vi "input.vi"(8 "error in":errorcluster, 10 "input allocation":T1, 11 "BuckBoost runtime in":refnum<class "BuckBoost runtime.lvclass">) -> (0 "error out":errorcluster, 2 "input data":T1, 3 "BuckBoost runtime out":refnum<class "BuckBoost runtime.lvclass">)   [LabVIEW 2017, in "BuckBoost runtime.lvclass"]
doc: "Provides an interface for reading data from a module at runtime. While this interface performs no operations, a child should provide an override which may read from any open sessions, references, or interfaces."
uses:
  BuckBoost runtime.lvclass
  <vilib>/NI/Tag Bus/table/data table.ctl
  input user data.ctl
  BuckBoost runtime.lvclass/BuckBoost runtime.ctl
  <vilib>/NI/PowerElectronicsControl/Buck-Boost/RealTime/BuckBoostInterface.lvlib
  <vilib>/NI/Tag Bus/table/data table.lvlib
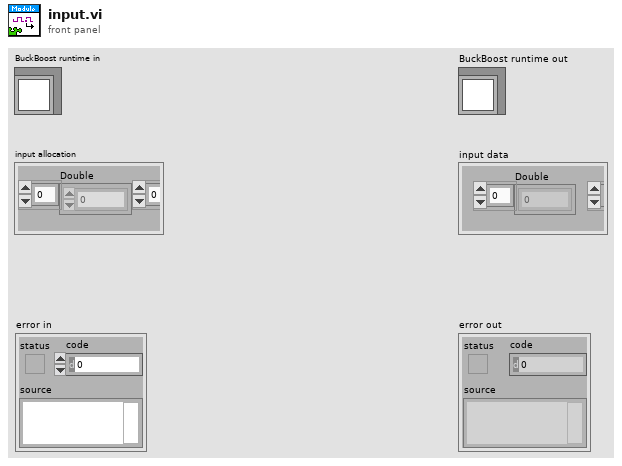
[diagram p1: front panel]
types:
  T1 = typedef "tag bus.lvlib/data table.lvlib/data table.ctl" = cluster{"Double":dbl[], "Single":sgl[], "I64":i64[], "I32":i32[], "I16":i16[], "I8":i8[], "U64":u64[], "U32":u32[], "U16":u16[], "U8":u8[], "Boolean":bool[], "String":string[], "Array of Double":cluster{"DBL Array":dbl[]}[], "Array of Single":cluster{"SGL Array":sgl[]}[], "Array of I64":cluster{"I64 Array":i64[]}[], "Array of I32":cluster{"I32 Array":i32[]}[], "Array of I16":cluster{"I16 Array":i16[]}[], "Array of I8":cluster{"I8 Array":i8[]}[], "Array of U64":cluster{"U64 Array":u64[]}[], "Array of U32":cluster{"U32 Array":u32[]}[], "Array of U16":cluster{"U16 Array":u16[]}[], "Array of U8":cluster{"U8 Array":u8[]}[], "Array of Boolean":cluster{"Boolean Array":bool[]}[], "Array of String":cluster{"String Array":string[]}[]}
  T2 = typedef "BuckBoost runtime.lvclass/input user data.ctl" = cluster{"Currents":dbl[], "Enabled":u8, "TotalCurrent":dbl}
  T3 = typedef "BuckBoost configuration.lvclass/input data indices.ctl" = cluster{"Array of Double.Currents":i32, "U8.Enabled":i32, "Double.TotalCurrent":i32}
  T4 = typedef "BuckBoostInterface.lvlib/Interface.ctl" = cluster{"instruction target":refnum<class "niInstr Instruction Target v1 Host.lvclass">, "BuckBoostContext":refnum<class "niInstr Instruction Framework Context v1 Host.lvclass">}
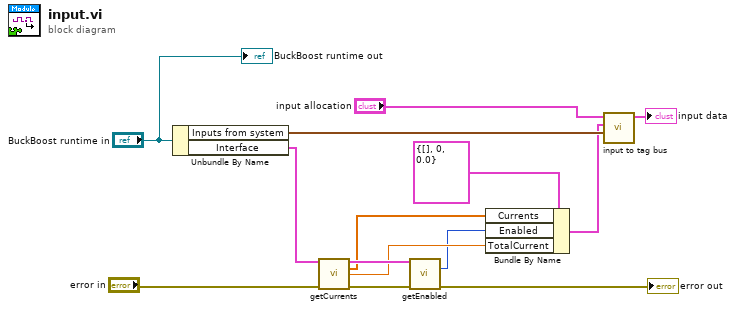
[diagram p0: block diagram]
diagram:
  n1 = Unbundle By Name("BuckBoost runtime in") -> ("Inputs from system"=w11:T3, "Interface"=w9:T4)
  n2 = call <vilib>:"getCurrents.vi"("Interface in"=w9, "error in (no error)"="error in") -> ("Interface out"=w8:T4, "Currents"=w4:sgl[], "TotalCurrent"=w3:sgl, "error out"=w7:errorcluster)  [unwired: 10 in]
  n3 = call <vilib>:"getEnabled.vi"("Interface in"=w8, "error in (no error)"=w7) -> ("Enabled"=w2:u8, "error out"=→"error out":errorcluster)  [unwired: 11 in, 1 out]
  n4 = Bundle By Name(cluster=T2 {"Currents"=[], "Enabled"=0, "TotalCurrent"=0.0} ("data cluster"), "Currents"=w4, "Enabled"=w2, "TotalCurrent"=w3) -> (w1:T2)
  n5 = call "input to tag bus.vi"("indices"=w11, "data cluster"=w1, "tag bus in"="input allocation") -> ("tag bus out"=→"input data":T1)  [unwired: 8 in]
  "BuckBoost runtime out" <- "BuckBoost runtime in"
